vi "wielomian.vi"() -> ()   [LabVIEW 2015]
panel:
  out "Waveform Chart":dbl(graph)
  out "Wynik":dbl
  in  "a0":dbl
  in  "a1":dbl
  in  "a2":dbl
  in  "a3":dbl
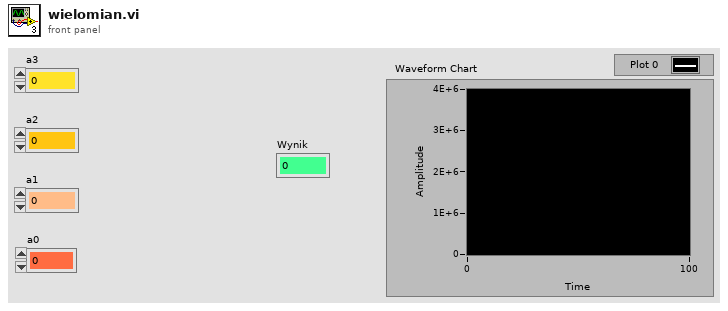
[diagram p1: front panel]
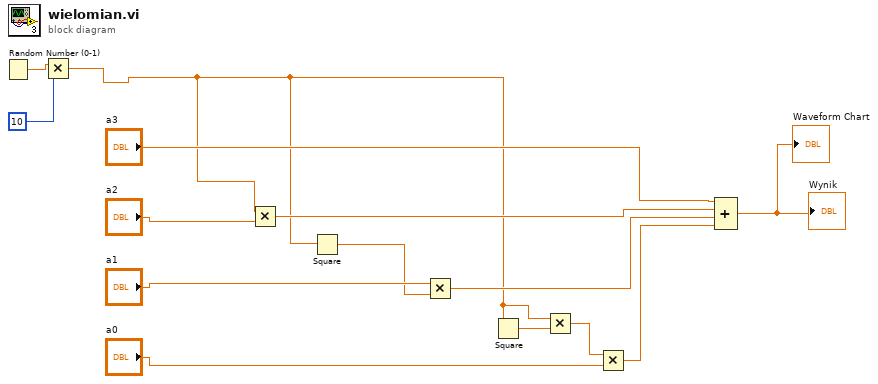
[diagram p0: block diagram]
diagram:
  n1 = Random Number (0-1)() -> (number: 0 to 1=w2:dbl)
  n2 = Multiply(x=w2, y=10) -> (x*y=w1:dbl)
  n3 = Multiply(x=w1, y="a2") -> (x*y=w11:dbl)
  n4 = Square(x=w1) -> (x^2=w7:dbl)
  n5 = Multiply(x="a1", y=w7) -> (x*y=w10:dbl)
  n6 = Square(x=w1) -> (x^2=w6:dbl)
  n7 = Multiply(x=w1, y=w6) -> (x*y=w5:dbl)
  n8 = Multiply(x=w5, y="a0") -> (x*y=w9:dbl)
  n9 = Compound Arithmetic op=ADD("a3", w11, w10, w9) -> (→"Wynik" →"Waveform Chart":dbl)
